vi "AddToScene.vi"(8 "error in (no error)":errorcluster, 10 "sceneRoot in":refnum<class "SceneRoot.lvclass">, 11 "class data in":refnum<class "SceneObject.lvclass">) -> (0 "error out":errorcluster, 3 "class data out":refnum<class "SceneObject.lvclass">)   [LabVIEW 2010, in "RenderBase.lvlib" / "SceneObject.lvclass"]
doc: "Adds the scene object to the given scene."
uses:
  SceneObject.lvclass
  SceneRoot_class/SceneRoot.lvclass
  SceneObject.lvclass/SceneObject.ctl
  SceneRoot_class/properties/Scene/GetScene.vi
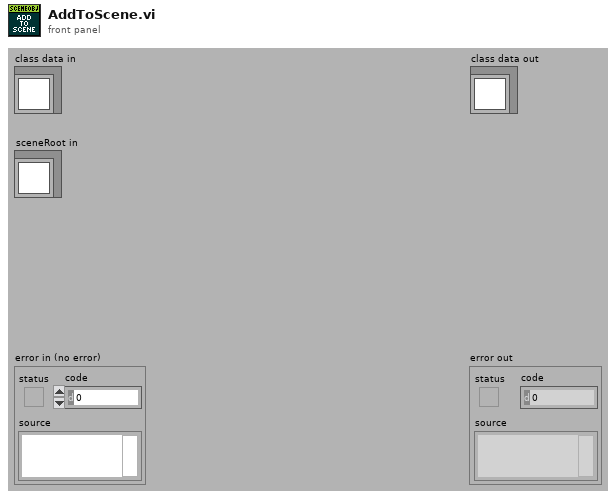
[diagram p1: front panel]
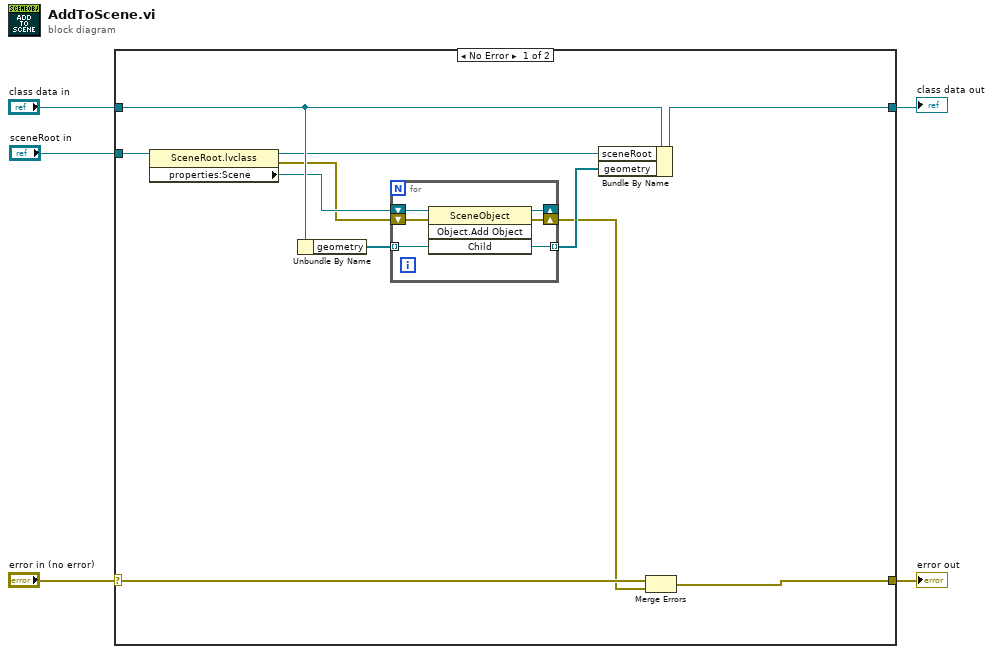
[diagram p0: block diagram]
diagram:
  n1 = case shown="No Error" "error in (no error)" {
    selector: "error in (no error)" -> [w16 w24]
    tunnel: [w7 w24] -> w4
    tunnel: "class data in" -> [w14 w23]
    tunnel: [w13 w23] -> w2
    tunnel: "sceneRoot in" -> [w12 _]
    frame No Error {
      n2 = property class="SceneRoot.lvclass"(reference=w12) -> (reference out=w11:refnum<class "SceneRoot.lvclass">, error out=w8:errorcluster, "properties:Scene"=w10:refnum<vi>)  [unwired: 1 in]
      n3 = Unbundle By Name(w14) -> ("geometry"=w15:refnum<vi>[])
      n4 = for {
        tunnel: w15 -> [w22] mode=indexing
        tunnel: [w20] -> w9 mode=indexing
        shift-right: [w19] -> _
        shift-left: w10 -> [w21]
        shift-right: [w17] -> w6
        shift-left: w8 -> [w18]
        n5 = invoke class="SceneObject" method="Object.Add Object"(reference=w21, error in=w18, "Child"=w22) -> (reference out=w19:refnum<vi>, error out=w17:errorcluster, "Child"=w20:refnum<vi>)  [unwired: 1 in, 1 out]
      }
      n6 = Bundle By Name(cluster=w14, "sceneRoot"=w11, "geometry"=w9) -> (w13:refnum<class "SceneObject.lvclass">)
      n7 = Merge Errors(w16, w6) -> (w7:errorcluster)
    }
    frame Error {
    }
  }
  "error out" <- w4
  "class data out" <- w2
